vi "Apply Theme.vi"(8 "error in":errorcluster, 11 "VI Refnum":refnum<vi>) -> (0 "error out":errorcluster)   [LabVIEW 2021]
doc: "Show this VI and let user define a new path/theme to apply to the VI.\n\n->Will be invoked with Quick Drop as a way to easily change the theme quickly during edit mode\n\n<b>Code Developed By:</b>\nTechnology Service Corporation\nwww.tsc.com/atcs\n\nDeveloper:\nDaniel Coons"
uses:
  Material Theme/Material Theme.lvclass
  user32.dll
panel:
  out "Name of VI":string
  in  "Theme":u16(ring) items=["Light", "Light Medium Contrast", "Light High Contrast", "Dark", "Dark Medium Contrast", "Dark High Contrast"]
  in  "done":bool
  out "header":bool
  in  "Path to theme file":path
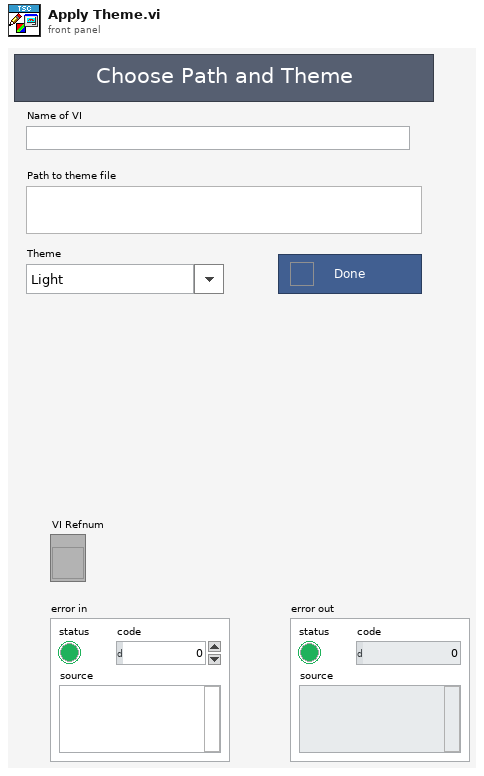
[diagram p1: front panel]
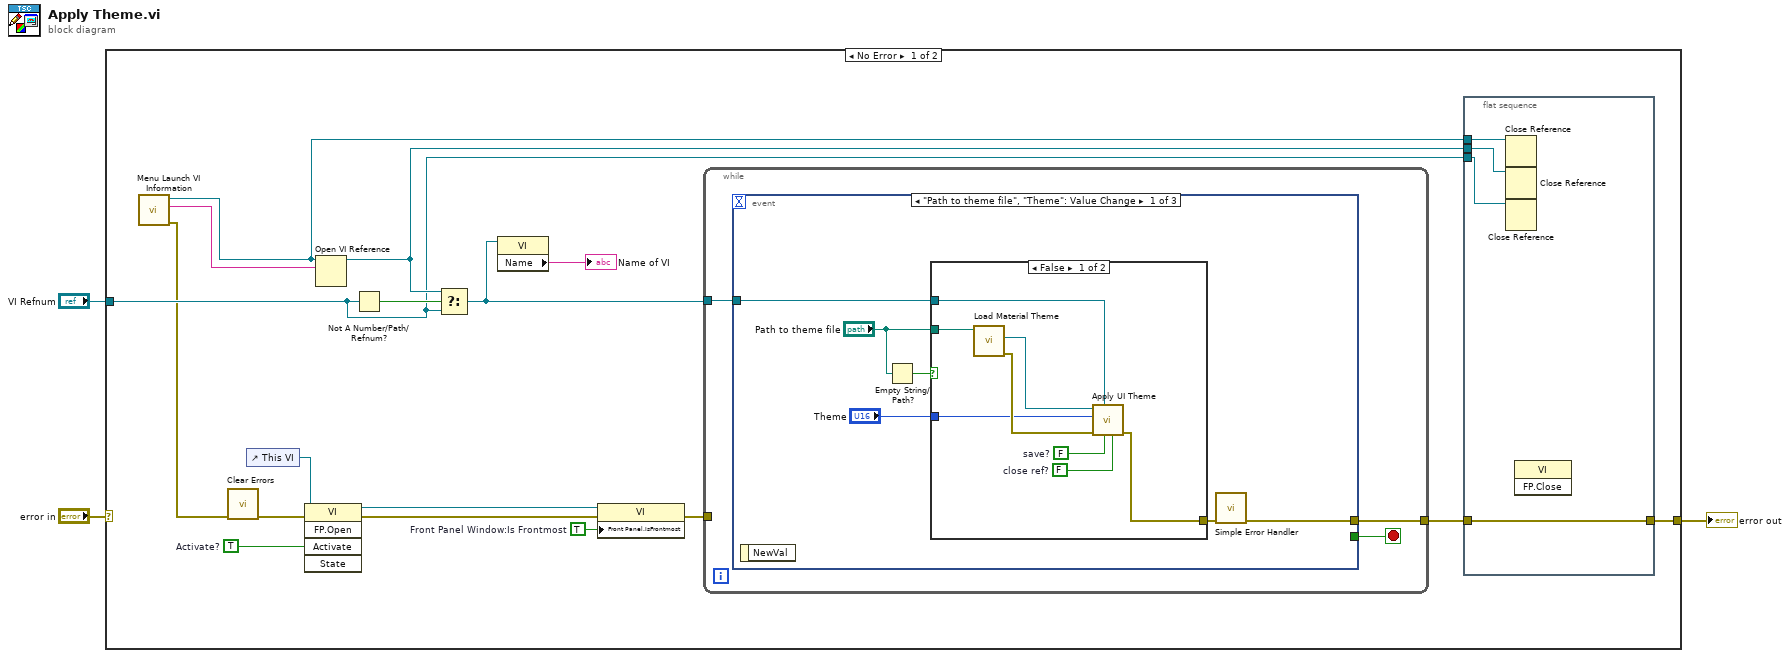
[diagram p0: block diagram]
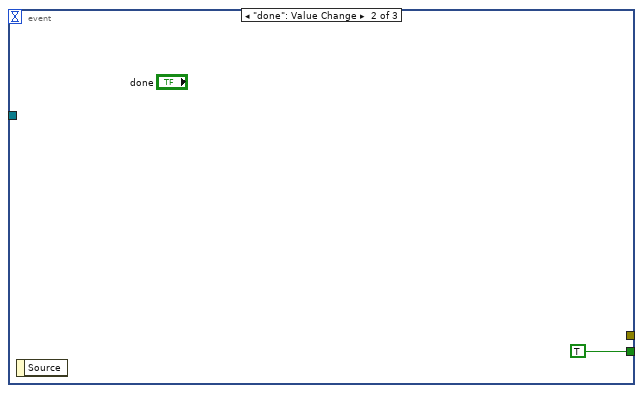
[diagram p3: hidden frame]
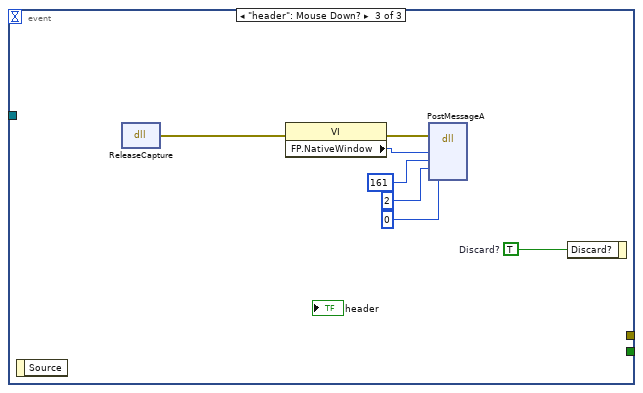
[diagram p4: hidden frame]
diagram:
  n1 = case shown="No Error" "error in" {
    selector: "error in" -> [_ w50]
    tunnel: "VI Refnum" -> [w9 _]
    tunnel: [w17 w50] -> w2
    frame No Error {
      w14 = TRUE  # Front Panel Window:Is Frontmost
      w19 = TRUE  # Activate?
      n2 = call <vilib>:"Menu Launch VI Information.vi"() -> ("error out"=w6:errorcluster, "Menu Launch:VI"=w7:string, "Menu Launch:App"=w8:refnum<vi>)  [unwired: 9 in]
      n3 = call <vilib>:"Clear Errors.vi"("error in (no error)"=w6) -> ("error out"=w4:errorcluster)  [unwired: 5 in, 1 out]
      n4 = control-ref of="This VI"() -> (w5:refnum<vi>)
      n5 = invoke class="VI" method="FP.Open"(reference=w5, error in=w4, "Activate"=w19) -> (reference out=w15:refnum<vi>, error out=w20:errorcluster)  [unwired: 2 in, 3 out]
      n6 = Open VI Reference(application reference (local)=w8, vi path=w7) -> (vi reference=w10:refnum<vi>)  [unwired: 4 in, 1 out]
      n7 = Not A Number/Path/Refnum?(number/path/refnum=w9) -> (NaN/Path/Refnum?=w13:bool)
      n8 = Select(t=w10, s=w13, f=w9) -> (s? t:f=w12:refnum<vi>)
      n9 = property class="VI"(reference=w12) -> ("Name"=→"Name of VI":string)  [unwired: 1 in, 2 out]
      n10 = property class="VI"(reference=w15, error in=w20, "Front Panel.IsFrontmost"=w14) -> (error out=w16:errorcluster)  [unwired: 1 out]
      n11 = while {
        tunnel: w12 -> [w27]
        tunnel: w16 -> [_]
        tunnel: [w26] -> w18
        stop <- w25 stop-if-true
        n12 = event shown="[0] \"Path to theme file\", \"Theme\": Value Change" {
          selector: _ -> [_ _ _]
          dyn-events: _ -> [_ _ _]
          timeout: _ -> [_ _ _]
          tunnel: w27 -> [w33 _ _]
          tunnel: [w31 _ _] -> w26
          tunnel: [_ TRUE _] -> w25
          event "Path to theme file", "Theme": Value Change {
            n13 = event-data() -> ()  [unwired: 1 in, 1 out]
            n14 = Empty String/Path?(string/path="Path to theme file") -> (empty?=w28:bool)
            n15 = case shown="False" w28 {
              tunnel: "Path to theme file" -> [w41 _]
              tunnel: w33 -> [w39 _]
              tunnel: [w37 _] -> w32
              tunnel: "Theme" -> [w34 _]
              frame False {
                w35 = FALSE  # save?
                w36 = FALSE  # close ref?
                n16 = call "Load Material Theme.vi"("file path (use dialog)"=w41) -> ("error out"=w38:errorcluster, "Theme"=w40:refnum<class "Material Theme.lvclass">)  [unwired: 9 in]
                n17 = call "Apply UI Theme.vi"("close ref?"=w36, "save?"=w35, "VI Refnum"=w39, "error in (no error)"=w38, "Theme"=w34, "Material Theme in"=w40) -> ("error out"=w37:errorcluster)  [unwired: 4 in, 1 out]
              }
              frame True {
              }
            }
            n18 = call <vilib>:"Simple Error Handler.vi"("error in (no error)"=w32) -> ("error out"=w31:errorcluster)  [unwired: 4 in, 4 out]
          }
          event "done": Value Change {
            n19 = event-data() -> ()  [unwired: 1 in, 1 out]
          }
          event "header": Mouse Down? {
            w49 = TRUE  # Discard?
            n20 = event-data() -> ()  [unwired: 1 in, 1 out]
            n21 = dll-call lib="user32.dll" fn="ReleaseCapture"() -> (error out=w45:errorcluster)  [unwired: 4 in, 1 out]
            n22 = property class="VI"(error in=w45) -> (error out=w44:errorcluster, "FP.NativeWindow"=w43:u64)  [unwired: 1 in, 1 out]
            n23 = dll-call lib="user32.dll" fn="PostMessageA"(error in=w44, "hWnd"=w43, "Msg"=161, "wParam"=2, "lParam"=0) -> ()  [unwired: 7 in, 2 out]
            n24 = event-data("Discard?"=w49) -> ()  [unwired: 1 in, 1 out]
          }
        }
      }
      n25 = flat-sequence {
        tunnel: w18 -> [w24]
        tunnel: [w24] -> w17
        tunnel: w8 -> [w23]
        tunnel: w10 -> [w22]
        tunnel: w9 -> [w21]
        frame #0 {
          n26 = Close Reference(reference=w23) -> ()  [unwired: 1 in, 1 out]
          n27 = Close Reference(reference=w22) -> ()  [unwired: 1 in, 1 out]
          n28 = Close Reference(reference=w21) -> ()  [unwired: 1 in, 1 out]
          n29 = invoke class="VI" method="FP.Close"() -> ()  [unwired: 3 in, 3 out]
        }
      }
    }
    frame Error {
    }
  }
  "error out" <- w2
